vi "Temperature_Bits_to_Deg.vi"(4 "TMax":dbl, 6 "TMin":dbl format="%#_13g", 11 "Val-In":dbl) -> (3 "TOut":dbl)   [LabVIEW 2021]
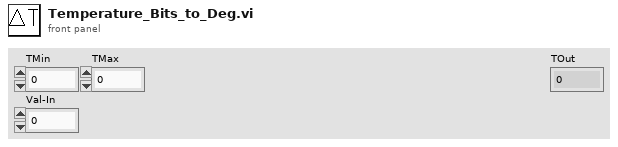
[diagram p1: front panel]
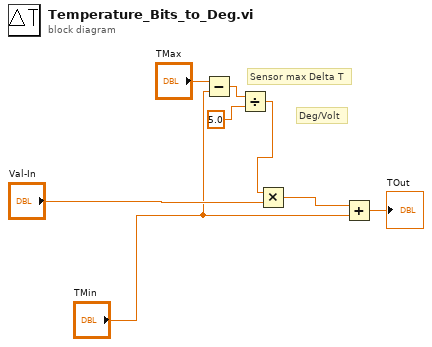
[diagram p0: block diagram]
diagram:
  # "Deg/Volt"
  # "Sensor max Delta T"
  n1 = Subtract(x="TMax", y="TMin") -> (x-y=w7:dbl)
  n2 = Divide(x=w7, y=5.0) -> (x/y=w5:dbl)
  n3 = Multiply(x=w5, y="Val-In") -> (x*y=w3:dbl)
  n4 = Add(x=w3, y="TMin") -> (x+y=→"TOut":dbl)
